vi "GetSpeed.vi"(8 "error in (no error)":errorcluster, 10 "Motor":T1, 11 "Map":T2) -> (0 "error out":errorcluster, 3 "Speed [RPM]":dbl=60.0)   [LabVIEW 2017, in "McsaAnalysisFunctions.lvlib"]
uses:
  <vilib>/addons/InsightCM/Utilities/Analysis/MCSA/McsaAnalysisFunctions.lvlib
  <vilib>/addons/PointValueMap/controls/PointMap.ctl
  <vilib>/addons/InsightCM/Utilities/Analysis/MCSA/controls/McsaMotor.ctl
  <vilib>/addons/PointValueMap/PointValueMap.lvlib
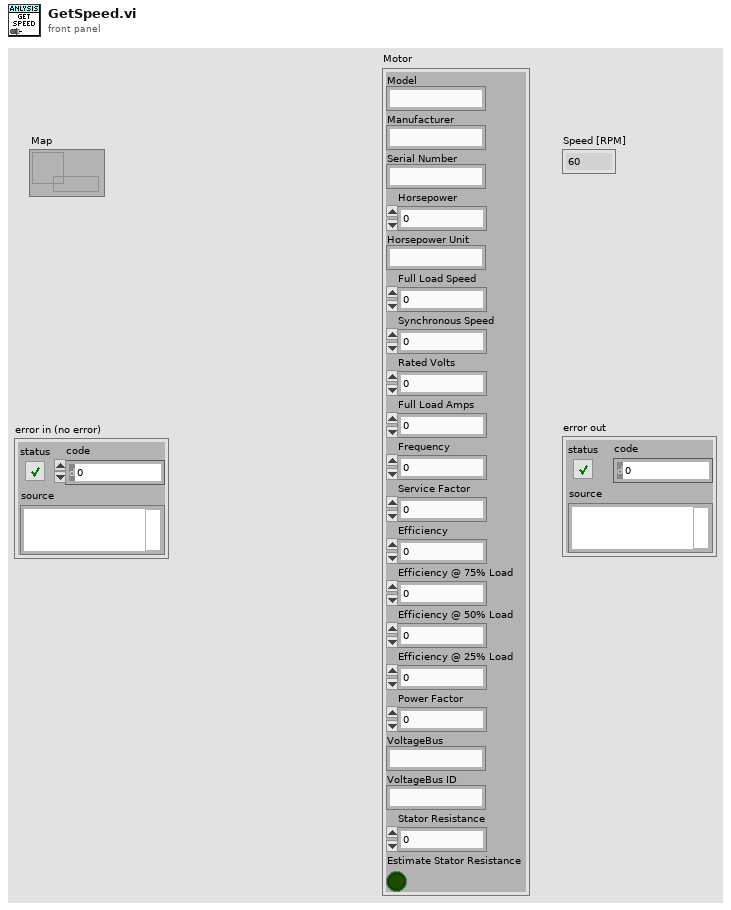
[diagram p1: front panel]
types:
  T1 = typedef "McsaAnalysisFunctions.lvlib/McsaMotor.ctl" = cluster{"Model":string, "Manufacturer":string, "Serial Number":string, "Horsepower":dbl, "Horsepower Unit":string, "Full Load Speed":dbl, "Synchronous Speed":dbl, "Rated Volts":dbl, "Full Load Amps":dbl, "Frequency":dbl, "Service Factor":dbl, "Efficiency":dbl, "Efficiency @ 75% Load":dbl, "Efficiency @ 50% Load":dbl, "Efficiency @ 25% Load":dbl, "Power Factor":dbl, "VoltageBus":string, "VoltageBus ID":string, "Stator Resistance":dbl, "Estimate Stator Resistance":bool}
  T2 = typedef "PointValueMap.lvlib/PointMap.ctl" = refnum<data-value>
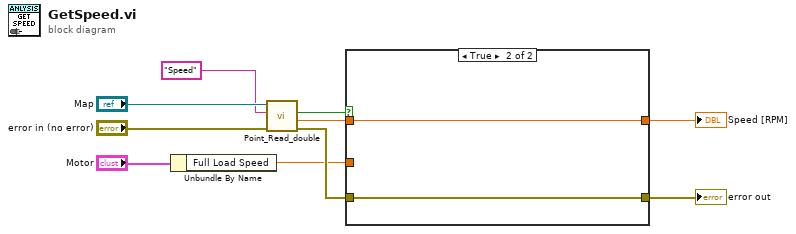
[diagram p0: block diagram]
diagram:
  n1 = Unbundle By Name("Motor") -> ("Full Load Speed"=w2:dbl)
  n2 = call <vilib>:"Point_Read_double.vi"("Error In"="error in (no error)", "Tag"="Speed", "Map"="Map") -> ("Error Out"=w5:errorcluster, "Value"=w4:dbl, "Found?"=w7:bool)  [unwired: 3 in, 3 out]
  n3 = case shown="True" w7 {
    tunnel: [w11 w13] -> w9
    tunnel: [w12 w14] -> w10
    tunnel: w5 -> [w12 w14]
    tunnel: w4 -> [_ w13]
    tunnel: w2 -> [w11 _]
    frame False {
    }
    frame True {
    }
  }
  "Speed [RPM]" <- w9
  "error out" <- w10
